vi "RS232ComPort ReadDeviceInfo.vi"(8 "error in (no error)":errorcluster, 9 "DeviceIndex":i32, 11 "RS232ComPort in":refnum<class "RS232ComPort.lvclass">) -> (0 "error out":errorcluster, 2 "DeviceInfo":T2, 3 "RS232ComPort out":refnum<class "RS232ComPort.lvclass">)   [LabVIEW 2018, in "RS232ComPort.lvclass"]
uses:
  RS232ComPort.lvclass
  RS232ComPort.lvclass/RS232ComPort.ctl
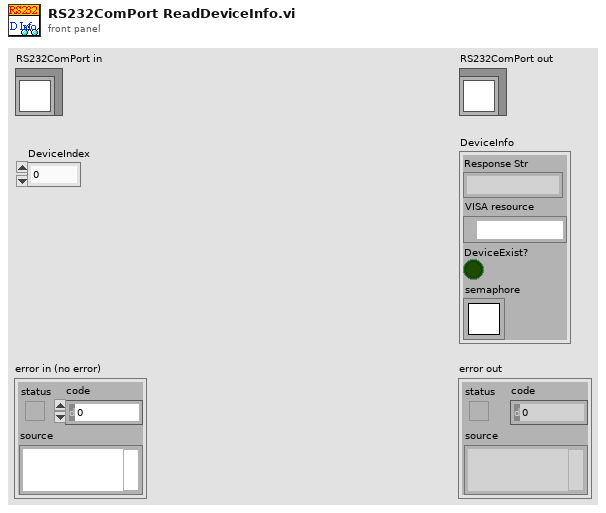
[diagram p1: front panel]
types:
  T1 = typedef "Semaphore RefNum" = refnum<k1>
  T2 = cluster{"Response Str":string, "VISA resource":refnum<visa-resource-name>, "DeviceExist?":bool, "semaphore":T1}
  T3 = cluster{"Response Str":string, "VISA resource":refnum<visa-resource-name>, "DeviceExist?":bool, "semaphore":T1}[]
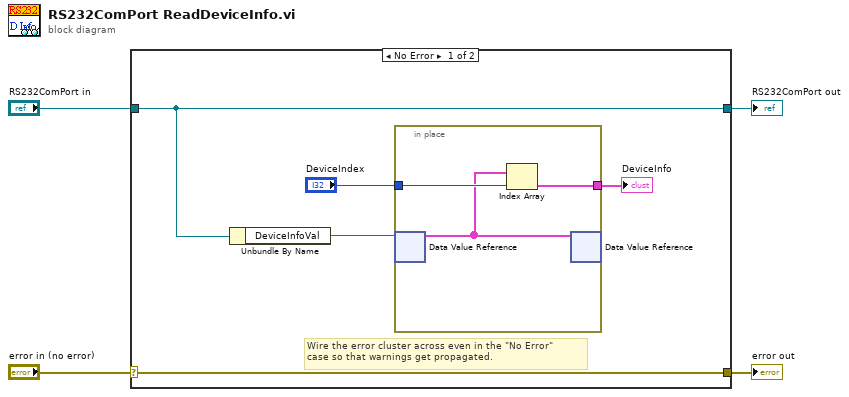
[diagram p0: block diagram]
diagram:
  n1 = case shown="No Error" "error in (no error)" {
    selector: "error in (no error)" -> [w9 w14]
    tunnel: [w9 w14] -> w3
    tunnel: [w8 w13] -> w1
    tunnel: "RS232ComPort in" -> [w8 w13]
    frame No Error {
      # "Wire the error cluster across even in the \"No Error\"\ncase so that warnings get propagated."
      n2 = Unbundle By Name(w8) -> ("DeviceInfoVal"=w7:refnum<data-value>)
      n3 = in-place {
        in-place-border: "DeviceIndex" -> [w12]
        in-place-border: [w10] -> w5
        n4 = in-place-dvr #1(w7) -> (w11:T3)  [unwired: 1 out]
        n5 = Index Array(array=w11, index=w12) -> (element=w10:T2)
        n6 = in-place-dvr #1(w11) -> ()  [unwired: 2 out]
      }
      "DeviceInfo" <- w5
    }
    frame Error {
    }
  }
  "error out" <- w3
  "RS232ComPort out" <- w1
